vi "AIP module.vi"(6 "Imaging Parameter.Line Averages":u8, 7 "Manual Controls.PSOCT Channel":u32, 8 "Y":i32=1100, 9 "X":i32=1100, 10 "Z":i32=100, 11 "3D volume":sgl[](array[numeric])) -> (2 "AIP":sgl[][](array[numeric]), 3 "Bline":dbl[][](array[numeric]))   [LabVIEW 2018]
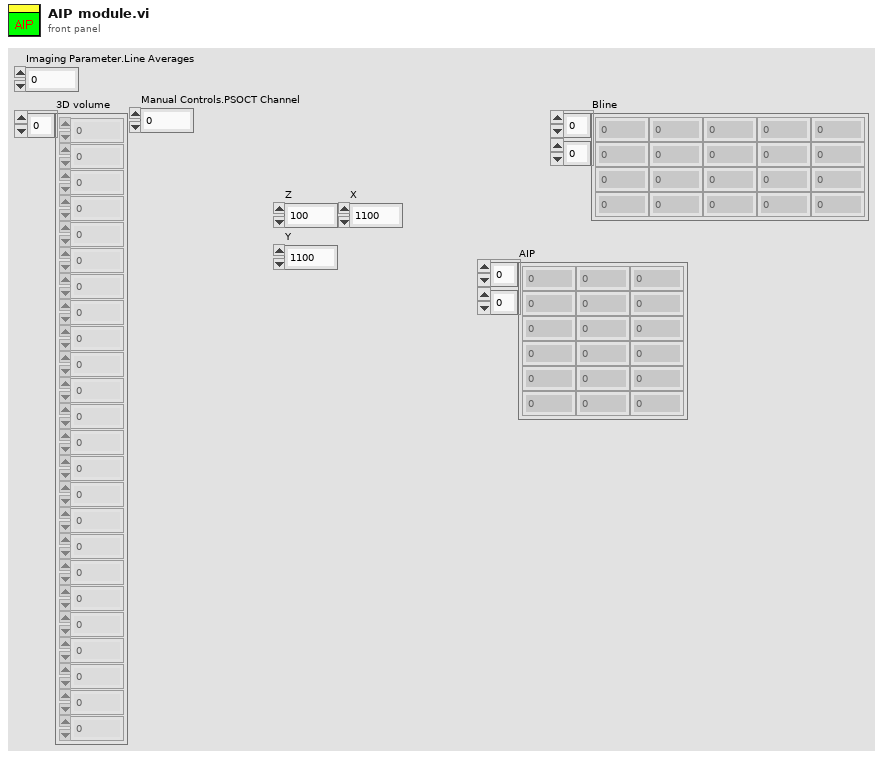
[diagram p1: front panel]
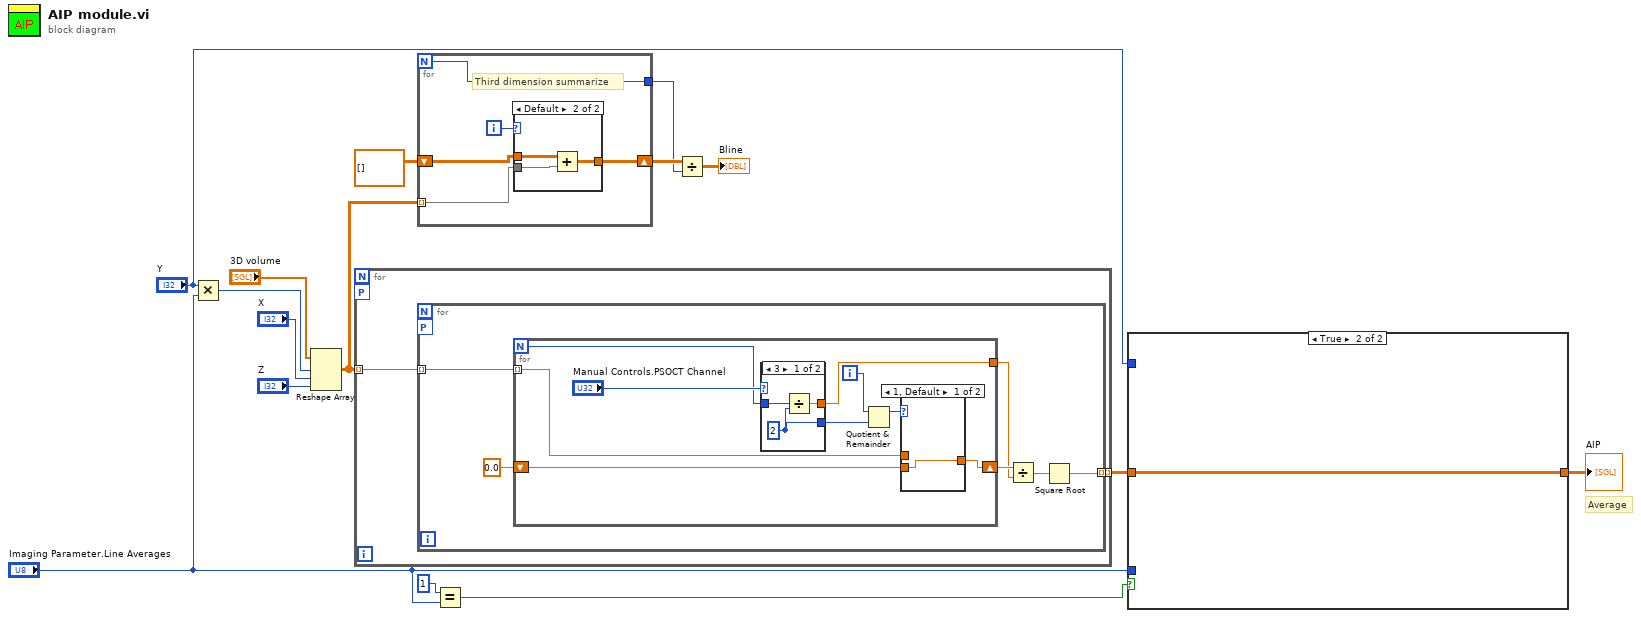
[diagram p0: block diagram]
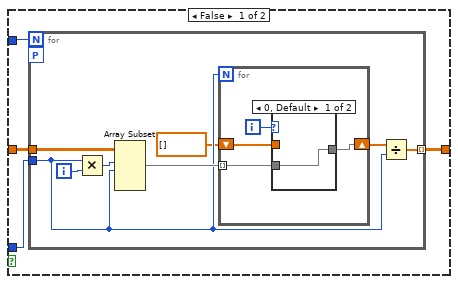
[diagram p2: hidden frame]
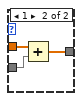
[diagram p3: hidden frame]
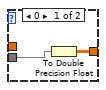
[diagram p4: hidden frame]
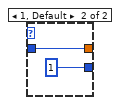
[diagram p5: hidden frame]
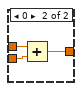
[diagram p6: hidden frame]
diagram:
  # "Average"
  n1 = Multiply(x="Y", y="Imaging Parameter.Line Averages") -> (x*y=w8:i32)
  n2 = Reshape Array("3D volume", w8, "X", "Z") -> (w1:sgl[][][])
  n3 = for {
    tunnel: w1 -> [w17] mode=indexing
    tunnel: [w16] -> w4 mode=indexing
    workers-P: _ -> [_]
    n4 = for {
      tunnel: w17 -> [w23] mode=indexing
      tunnel: [w18] -> w16 mode=indexing
      workers-P: _ -> [_]
      n5 = for {
        N -> [w25]
        tunnel: w23 -> [w32] mode=indexing
        shift-right: [w30] -> w22
        shift-left: sgl 0.0 -> [w31]
        tunnel: [w24] -> w21
        i -> [w29]
        n6 = case shown="3" "Manual Controls.PSOCT Channel" {
          tunnel: [w35 1 ("y")] -> w28
          tunnel: w25 -> [w34 w36]
          tunnel: [w33 w36] -> w24
          frame 3 {
            w35 = 2 ("y")
            n7 = Divide(x=w34, y=w35) -> (x/y=w33:dbl)
          }
          frame 1, Default {
          }
        }
        n8 = Quotient & Remainder(x=w29, y=w28) -> (x-y*floor(x/y)=w27:i32)  [unwired: 1 out]
        n9 = case shown="1, Default" w27 {
          tunnel: w32 -> [_ w41]
          tunnel: w31 -> [w38 w40]
          tunnel: [w38 w39] -> w30
          frame 1, Default {
          }
          frame 0 {
            n10 = Add(x=w41, y=w40) -> (x+y=w39:sgl)
          }
        }
      }
      n11 = Divide(x=w22, y=w21) -> (x/y=w19:dbl)
      n12 = Square Root(x=w19) -> (sqrt(x)=w18:dbl)
    }
  }
  n13 = for {
    N -> [w43]
    shift-right: [w46] -> w11
    shift-left: sgl[][] [] -> [w45]
    tunnel: [w43] -> w10
    tunnel: w1 -> [w42] mode=indexing
    i -> [w44]
    # "Third dimension summarize"
    n14 = case shown="Default" w44 {
      tunnel: [w48 w51] -> w46
      tunnel: w45 -> [_ w50]
      tunnel: w42 -> [w47 w49]
      frame 0 {
        n15 = To Double Precision Float(number=w47) -> (double precision float=w48:dbl[][])
      }
      frame Default {
        n16 = Add(x=w50, y=w49) -> (x+y=w51:dbl[][])
      }
    }
  }
  n17 = Equal?(x=u8 1, y="Imaging Parameter.Line Averages") -> (x = y?=w7:bool)
  n18 = Divide(x=w11, y=w10) -> (x/y=→"Bline":dbl[][])
  n19 = case shown="True" w7 {
    tunnel: [w52 w72] -> w5
    tunnel: w4 -> [w55 w72]
    tunnel: "Y" -> [w54 _]
    tunnel: "Imaging Parameter.Line Averages" -> [w53 _]
    frame False {
      n20 = for {
        N: w54 -> [_]
        tunnel: w55 -> [w62]
        tunnel: w53 -> [w58]
        tunnel: [w57] -> w52 mode=indexing
        workers-P: _ -> [_]
        i -> [w63]
        n21 = Multiply(x=w58, y=w63) -> (x*y=w61:i32)
        n22 = Array Subset(array=w62, index (row)=w61, length (row)=w58) -> (w60:dbl[][])  [unwired: 2 in]
        n23 = for {
          N: w58 -> [_]
          tunnel: w60 -> [w66] mode=indexing
          shift-right: [w65] -> w59
          shift-left: sgl[] [] -> [w64]
          i -> [w67]
          n24 = case shown="0, Default" w67 {
            tunnel: w66 -> [w68 w71]
            tunnel: [w68 w70] -> w65
            tunnel: w64 -> [_ w69]
            frame 0, Default {
            }
            frame 1 {
              n25 = Add(x=w69, y=w71) -> (x+y=w70:dbl[])
            }
          }
        }
        n26 = Divide(x=w59, y=w58) -> (x/y=w57:dbl[])
      }
    }
    frame True {
    }
  }
  "AIP" <- w5
